vi "AWS Credentials Dialog.vi"(8 "error in (no error)":errorcluster) -> (0 "error out":errorcluster, 2 "Secret Access Key":string="fpHFy/9MTHgVK4Kfo+TPLrNeMAvaW8SEbrhzqAeY", 3 "Access Key ID":string="AKIAZ3CRVRJNHJHHHPO3")   [LabVIEW 2019, in "LV-Data.S3.lvclass"]
uses:
  LV-Data.S3.lvclass
  <vilib>/Platform/browser.llb/Open URL in Default Browser (string).vi
panel:
  in  "Message":string="Please enter your AWS credentials below:"
  in  "OK":bool caption="OK1"
  in  "HELP":bool caption="OK1"
  in  "Secret Access Key":string
  in  "Access Key ID":string
  out "String":string="Please enter your AWS credentials below:"
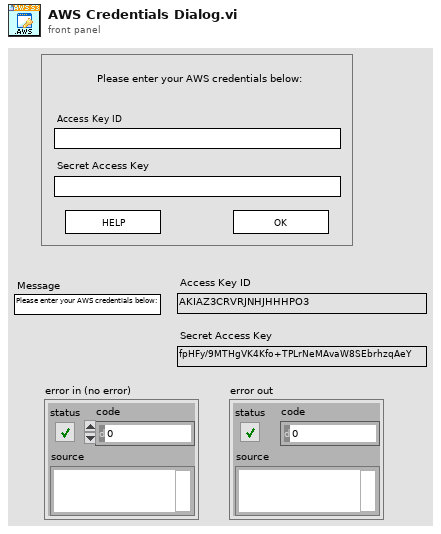
[diagram p1: front panel]
types:
  T1 = enum32{"Invalid", "Standard", "Closed", "Hidden", "Minimized", "Maximized"}
  T2 = enum32{"invalid app kind", "Development System", "Run Time System", "Student Edition", "Embedded LabVIEW", "Evaluation", "Custom"}
  T3 = cluster{"Core":cluster{"Current VI Reference":refnum<vi>, "Close Panel on Exit?":bool}, "Access Key ID":string, "Secret Access Key":string}
  T4 = cluster{"Current VI Reference":refnum<vi>, "Close Panel on Exit?":bool}
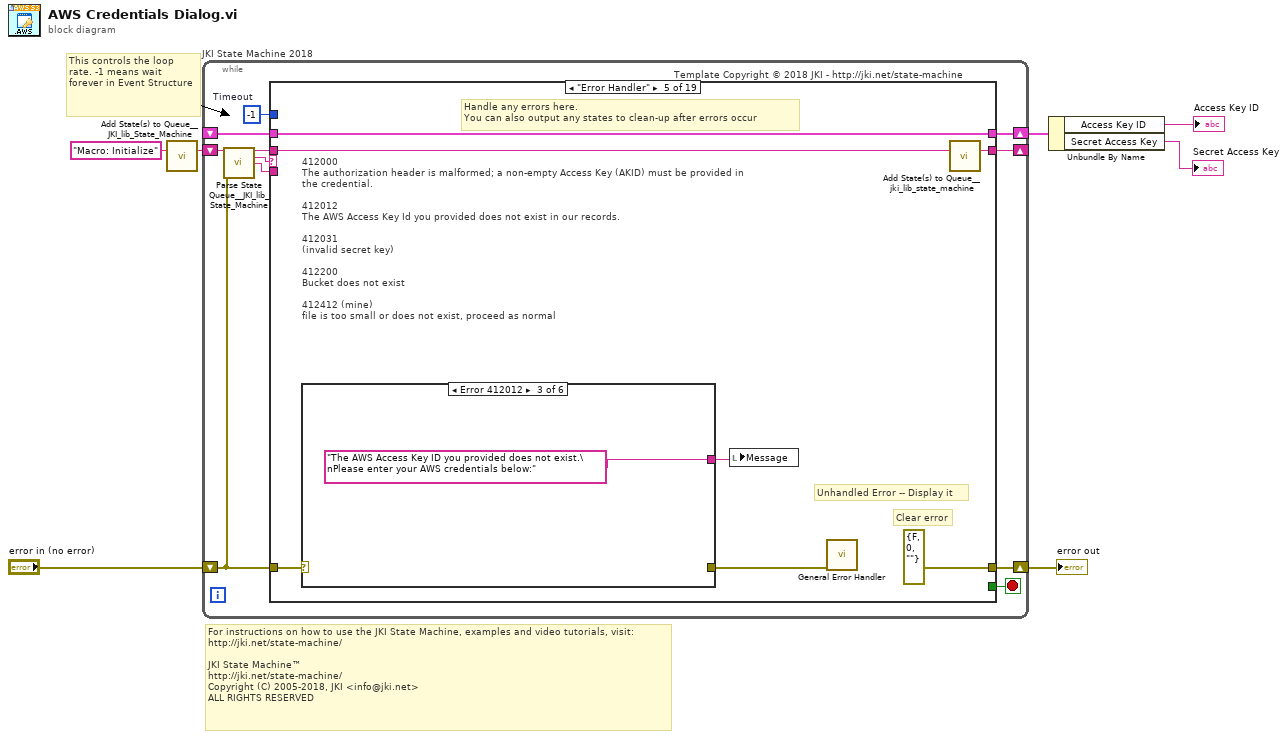
[diagram p0: block diagram]
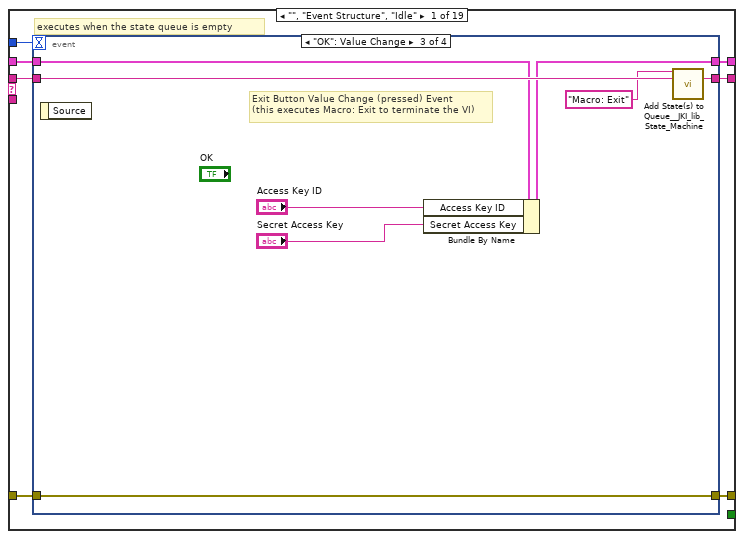
[diagram p2: hidden frame]
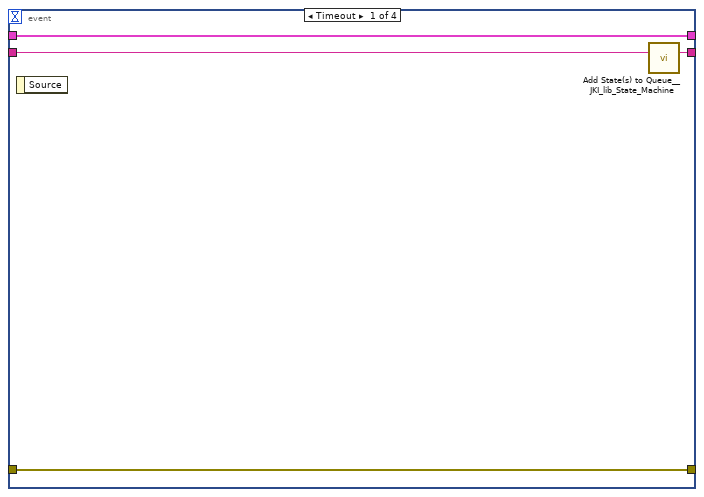
[diagram p3: hidden frame]
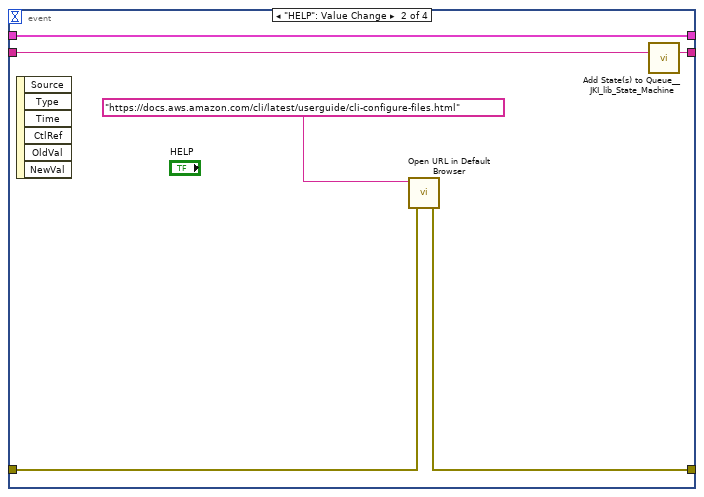
[diagram p4: hidden frame]
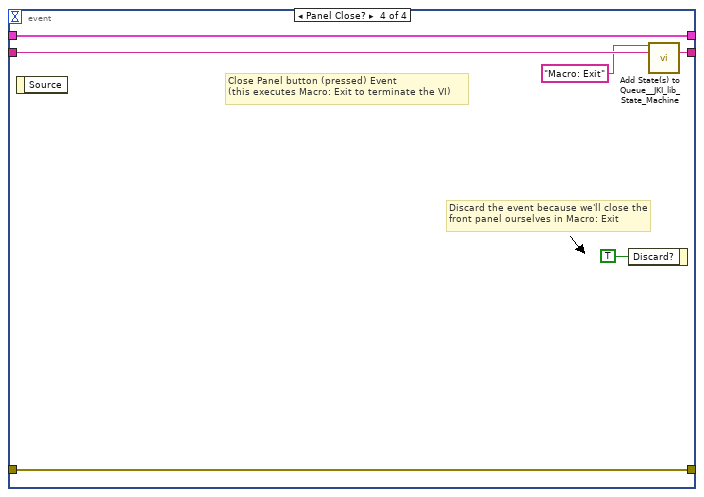
[diagram p5: hidden frame]
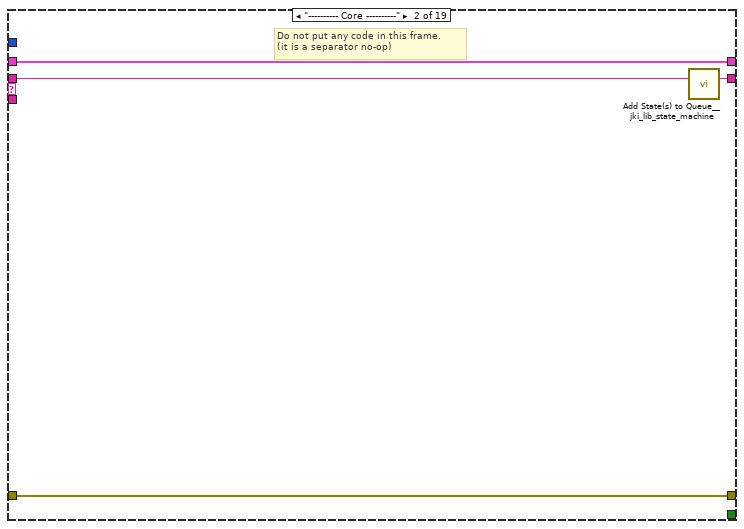
[diagram p6: hidden frame]
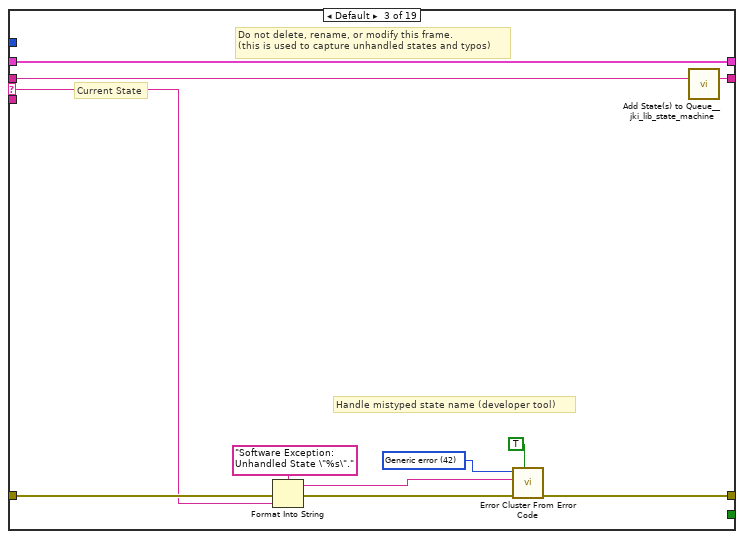
[diagram p7: hidden frame]
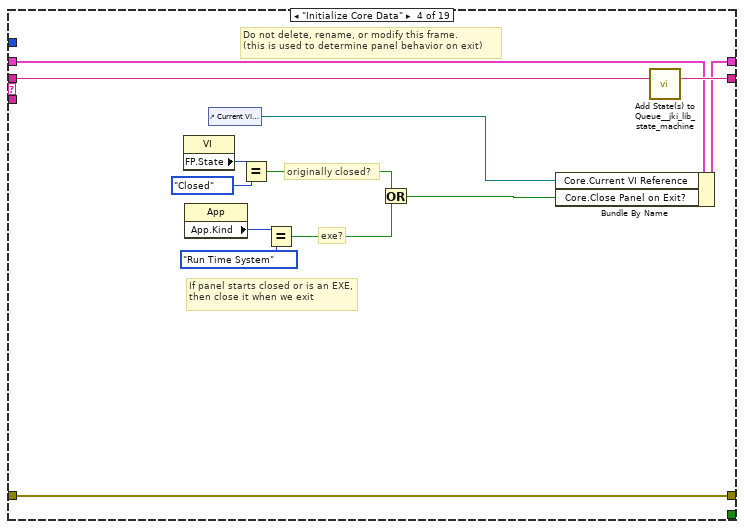
[diagram p8: hidden frame]
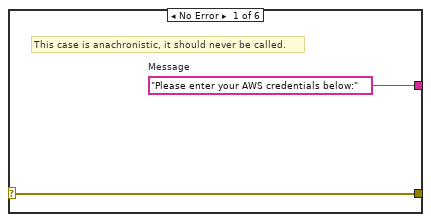
[diagram p9: hidden frame]
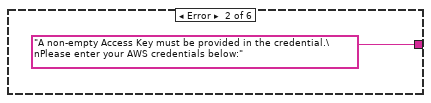
[diagram p10: hidden frame]
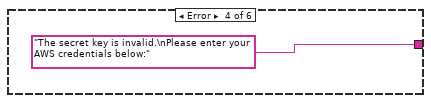
[diagram p11: hidden frame]
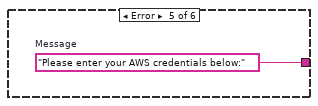
[diagram p12: hidden frame]
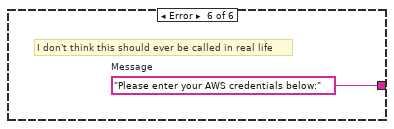
[diagram p13: hidden frame]
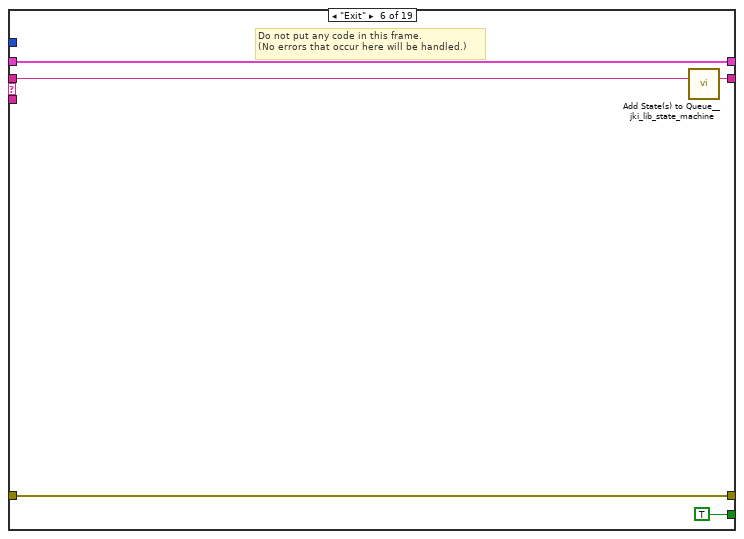
[diagram p14: hidden frame]
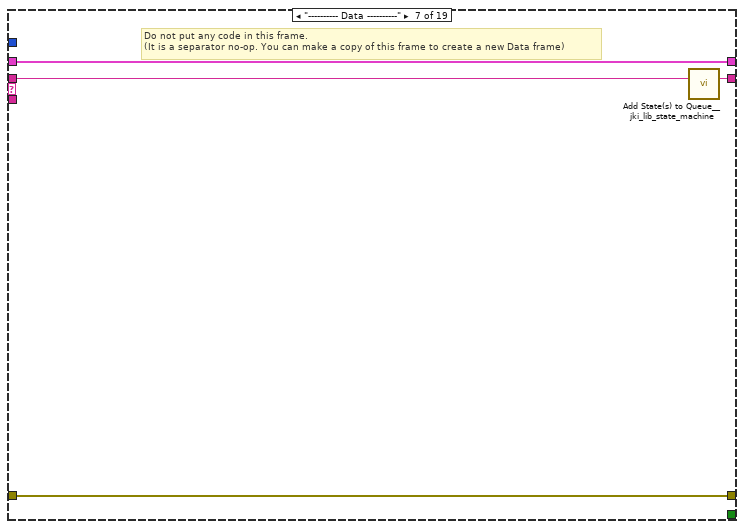
[diagram p15: hidden frame]
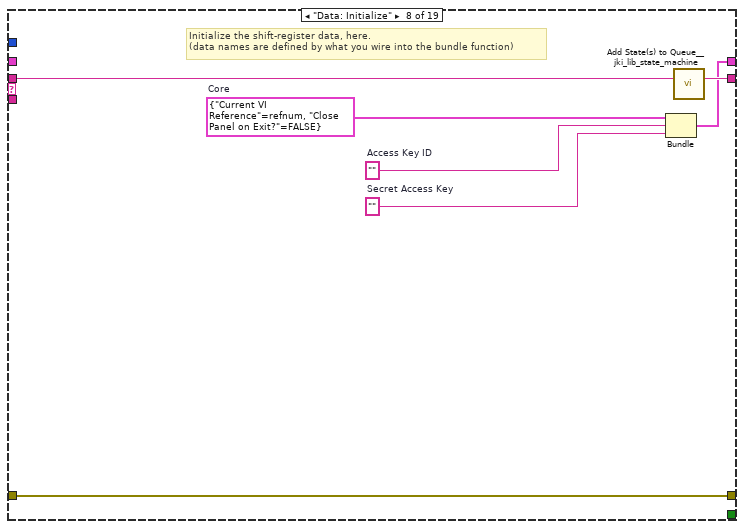
[diagram p16: hidden frame]
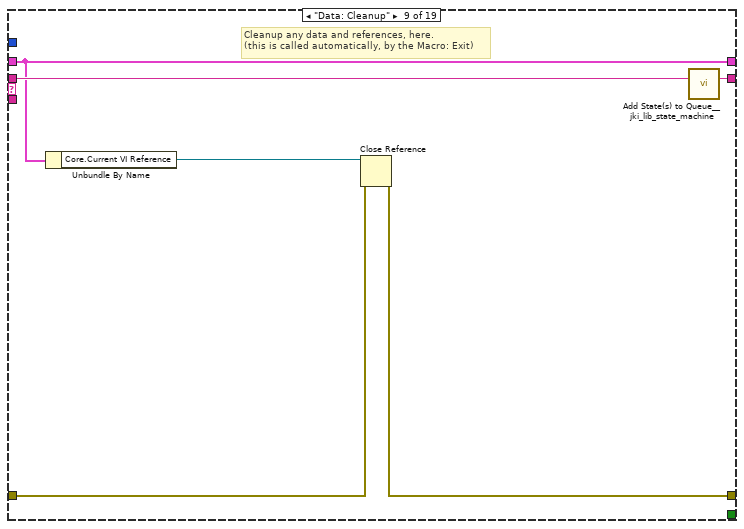
[diagram p17: hidden frame]
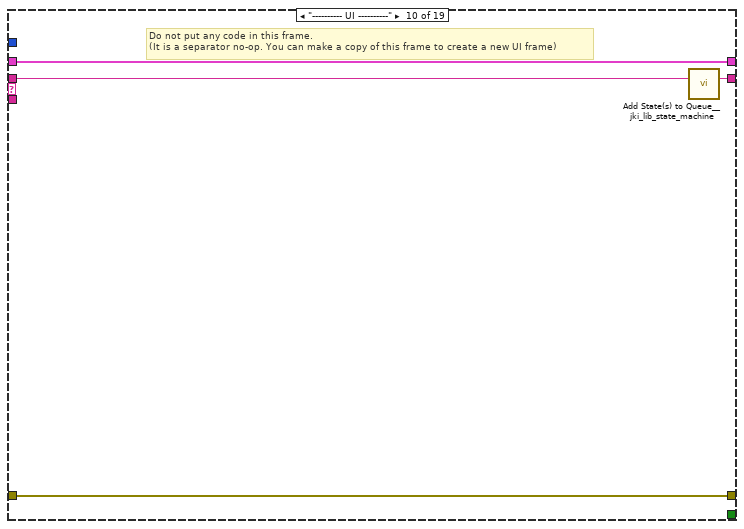
[diagram p18: hidden frame]
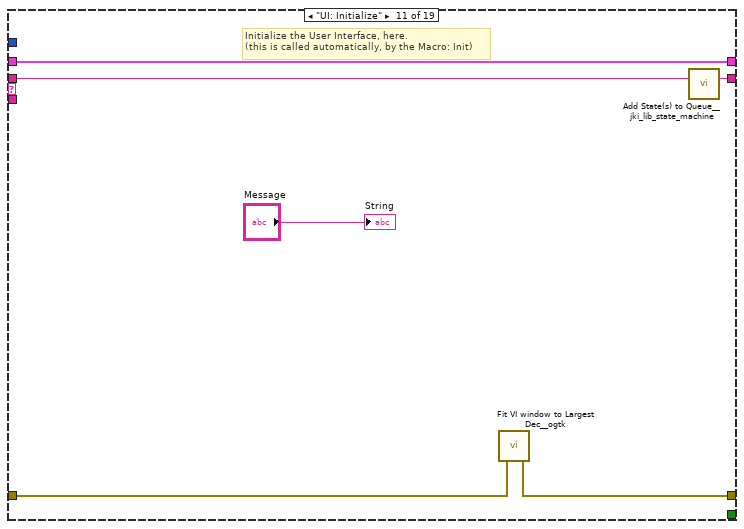
[diagram p19: hidden frame]
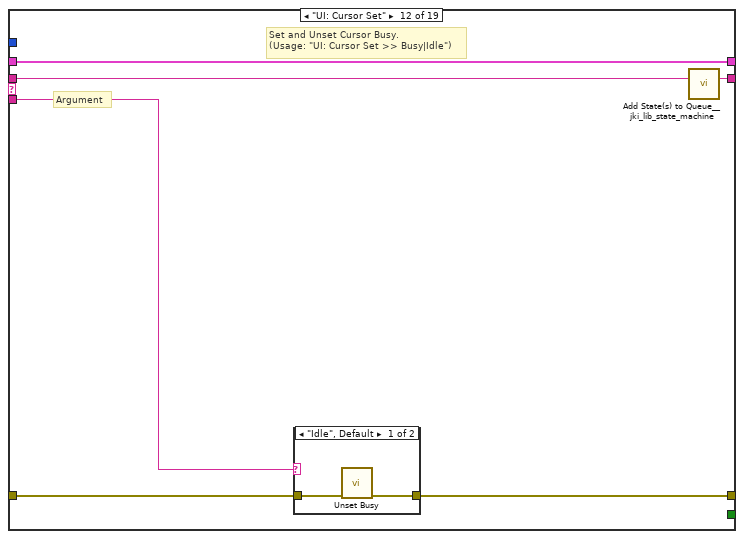
[diagram p20: hidden frame]
diagram:
  # "For instructions on how to use the JKI State Machine, examples and video tutorials, visit:\nhttp://jki.net/state-machine/\n\nJKI State Machine™\nhttp://jki.net/state-machine/\nCopyright (C) 2005-2018, JKI <info@jki.net>\nALL RIGHTS RESERVED"
  # "This controls the loop rate. -1 means wait forever in Event Structure"
  n1 = call <vilib>:"Add State(s) to Queue__JKI_lib_State_Machine.vi"("State(s) in (\"\")"="Macro: Initialize") -> ("States Out"=w7:string)  [unwired: 14 in]
  n2 = while "JKI State Machine 2018" {
    shift-right: [w11] -> w3
    shift-left: _ -> [w10]
    shift-right: [w14] -> w5
    shift-left: "error in (no error)" -> [w8]
    shift-right: [w13] -> _
    shift-left: w7 -> [w15]
    stop <- w12 stop-if-true
    w9 = -1  # Timeout
    # "Template Copyright © 2018 JKI - http://jki.net/state-machine"
    n3 = call <vilib>:"Parse State Queue__JKI_lib_State_Machine.vi"("State Queue"=w15, "Error In (no error)"=w8) -> ("Remaining States"=w17:string, "Current State"=w18:string, "Arguments"=w16:string)  [unwired: 11 in]
    n4 = case shown="\"Error Handler\"" w18 {
      selector: w18 -> [_ _ w54 _ _ _ _ _ _ _ _ _ _ _ _ _ _ _ _]
      tunnel: w17 -> [w25 w53 w58 w77 w84 w96 w100 w107 w113 w117 w123 w129 w140 w209 w214 w224 w228 w232 w236]
      tunnel: w16 -> [_ _ _ _ _ _ _ _ _ _ _ w124 w134 _ _ _ _ _ _]
      tunnel: w10 -> [w23 w50 w56 w70 w78 w94 w97 _ w108 w114 w121 w127 w136 w206 w211 w221 w225 w229 w233]
      tunnel: [w22 w51 w60 w74 errorcluster {"status"=FALSE, "code"=0, "source"=""} ("error out") w93 w98 w104 w109 w115 w119 w125 w137 w207 w212 w222 w226 w230 w234] -> w14
      tunnel: w8 -> [w21 w51 w59 w74 w81 w93 w98 w104 w110 w115 w120 w126 w138 w207 w212 w222 w226 w230 w234]
      tunnel: [w24 w52 w57 w76 w83 w95 w99 w106 w112 w116 w122 w128 w139 w208 w213 w223 w227 w231 w235] -> w13
      tunnel: [_ _ _ _ _ TRUE _ _ _ _ _ _ _ _ _ _ _ _ _] -> w12
      tunnel: [w20 w50 w56 w75 w78 w94 w97 w105 w108 w114 w121 w127 w136 w206 w211 w221 w225 w229 w233] -> w11
      tunnel: w9 -> [w19 _ _ _ _ _ _ _ _ _ _ _ _ _ _ _ _ _ _]
      frame "", "Event Structure", "Idle" {
        # "executes when the state queue is empty"
        n5 = event shown="[2] \"OK\": Value Change" {
          selector: _ -> [_ _ _ _]
          dyn-events: _ -> [_ _ _ _]
          timeout: w19 -> [_ _ _ _]
          tunnel: w25 -> [w29 w35 w43 w49]
          tunnel: [w28 w34 w42 w48] -> w24
          tunnel: w23 -> [w26 w33 w39 w46]
          tunnel: [w27 w31 w41 w47] -> w22
          tunnel: w21 -> [w27 w32 w41 w47]
          tunnel: [w26 w33 w38 w46] -> w20
          event Timeout {
            n6 = event-data() -> ()  [unwired: 1 in, 1 out]
            n7 = call <vilib>:"Add State(s) to Queue__JKI_lib_State_Machine.vi"("State(s) in (\"\")"=w29) -> ("States Out"=w28:string)  [unwired: 14 in]
          }
          event "HELP": Value Change {
            n8 = event-data() -> ()  [unwired: 1 in, 6 out]
            n9 = call-poly <vilib>:"Open URL in Default Browser.vi"("error in (no error)"=w32, "URL"="https://docs.aws.amazon.com/cli/latest/userguide/cli-configure-files.html") -> ("error out"=w31:errorcluster)  [unwired: 4 in, 1 out]
            n10 = call <vilib>:"Add State(s) to Queue__JKI_lib_State_Machine.vi"("State(s) in (\"\")"=w35) -> ("States Out"=w34:string)  [unwired: 14 in]
          }
          event "OK": Value Change {
            # "Exit Button Value Change (pressed) Event\n(this executes Macro: Exit to terminate the VI)"
            n11 = event-data() -> ()  [unwired: 1 in, 1 out]
            n12 = Bundle By Name(cluster=w39, "Access Key ID"="Access Key ID", "Secret Access Key"="Secret Access Key") -> (w38:T3)
            n13 = call <vilib>:"Add State(s) to Queue__JKI_lib_State_Machine.vi"("State(s) in Front (\"\")"="Macro: Exit", "State(s) in (\"\")"=w43) -> ("States Out"=w42:string)  [unwired: 13 in]
          }
          event Panel Close? {
            # "Discard the event because we'll close the front panel ourselves in Macro: Exit"
            # "Close Panel button (pressed) Event\n(this executes Macro: Exit to terminate the VI)"
            n14 = event-data() -> ()  [unwired: 1 in, 1 out]
            n15 = event-data("Discard?"=TRUE) -> ()  [unwired: 1 in, 1 out]
            n16 = call <vilib>:"Add State(s) to Queue__JKI_lib_State_Machine.vi"("State(s) in Front (\"\")"="Macro: Exit", "State(s) in (\"\")"=w49) -> ("States Out"=w48:string)  [unwired: 13 in]
          }
        }
      }
      frame "---------- Core ----------" {
        # "Do not put any code in this frame.\n(it is a separator no-op)"
        n17 = call <vilib>:"Add State(s) to Queue__jki_lib_state_machine.vi"("State(s) in (\"\")"=w53) -> ("States Out"=w52:string)  [unwired: 14 in]
      }
      frame Default {
        w63 = 42 items=["No error", "Argument error", "Memory is full", "Out of zone", "End of file", "File already open", "Generic file I/O error", "File not found", "File permission error", "Disk is full", "Duplicate path", "Too many files open", "System feature not enabled", "Resource file not found", "Cannot add resource", "Resource not found", "Image not found", "Image memory error", "Pen does not exist", "Config type invalid", "Config token not found", "Config parse error", "Config memory error", "Bad external code format", "Bad external code offset", "External code not present", "Null window", "Destroy window error", "Null menu", "Print aborted", "Bad print record", "Print driver error", "Windows error during printing", "Memory error during printing", "Print dialog error", "Generic print error", "Invalid device refnum", "Device not found", "Device parameter error", "Device unit error", "Cannot open device", "Device call aborted", "Generic error", "Cancelled by user", "Object ID too low", "Object ID too high", "Object not in heap", "Unknown heap", "Unknown object (invalid DefProc)", "Unknown object (DefProc not in table)", "Message out of range", "Invalid (null) method", "Unknown message", "Manager call not supported", "Bad address", "Network operation in progress", "Network operation timed out", "Connection is busy", "Network attribute not supported", "Network error", "Address in use", "System out of memory", "Connection aborted", "Connection refused", "Not connected", "Already connected", "Connection closed", "Initialization error (interapplication manager)", "Bad occurrence", "Wait on unbound occurrence handler", "Occurrence queue overflow", "Datalog type conflict", "Unused", "Unrecognized type (interapplication manager)", "Memory corrupt", "Failed to make temporary DLL", "Old CIN version", "Drag socket not found", "Failed to load drop-object", "Failed to register OLE object", "Failed to release OLE object", "Format specifier type mismatch", "Unknown format specifier", "Too few format specifiers", "Too many format specifiers", "Scan failed", "Newer CIN version", "Error converting to variant", "Runtime menu error", "Password tampered", "Variant attribute not found", "Incompatible variant data type", "Event data is not available", "Event Store is not present", "Occurrence is not found", "Event Queue is not created", "Event info is not available", "Refnum passed is NULL", "Error retrieving Class GUID", "Error retrieving CoClass GUID", "Error retrieving TypeLib GUID.", "Bad built application magic bytes.", "Specific driver is different from the specific driver associated with the Logical Name.", "There is no session opened to the class driver.", "Max Error", "MAX - Error with config objects", "MAX - Error loading configuration", "MAX - Group not supported"]
        # "Current State"
        # "Do not delete, rename, or modify this frame.\n(this is used to capture unhandled states and typos)"
        # "Handle mistyped state name (developer tool)"
        n18 = Format Into String(format string="Software Exception: Unhandled State \"%s\"." ("message"), error in=w59, w54) -> (resulting string=w62:string, error out=w61:errorcluster)  [unwired: 1 in]
        n19 = call <vilib>:"Error Cluster From Error Code.vi"("show call chain? (False)"=TRUE, "error in (no error)"=w61, "error message (\"\")"=w62, "error code (0)"=w63) -> ("error out"=w60:errorcluster)  [unwired: 5 in]
        n20 = call <vilib>:"Add State(s) to Queue__jki_lib_state_machine.vi"("State(s) in (\"\")"=w58) -> ("States Out"=w57:string)  [unwired: 14 in]
      }
      frame "Initialize Core Data" {
        # "Do not delete, rename, or modify this frame.\n(this is used to determine panel behavior on exit)"
        # "originally closed?"
        # "exe?"
        # "If panel starts closed or is an EXE, then close it when we exit"
        n21 = property class="VI"() -> ("FP.State"=w67:T1)  [unwired: 2 in, 2 out]
        n22 = property class="App"() -> ("App.Kind"=w73:T2)  [unwired: 2 in, 2 out]
        n23 = control-ref of="Current VI Reference"() -> (w68:refnum<vi>)
        n24 = Equal?(x=w67, y=T1."Closed" ("Front Panel Window:State")) -> (x = y?=w65:bool)
        n25 = Equal?(x=w73, y=T2."Run Time System" ("Application:Kind")) -> (x = y?=w71:bool)
        n26 = Or(x=w65, y=w71) -> (x .or. y?=w69:bool)
        n27 = Bundle By Name(cluster=w70, "Core.Current VI Reference"=w68, "Core.Close Panel on Exit?"=w69) -> (w75:T3)
        n28 = call <vilib>:"Add State(s) to Queue__jki_lib_state_machine.vi"("State(s) in (\"\")"=w77) -> ("States Out"=w76:string)  [unwired: 14 in]
      }
      frame "Error Handler" {
        # "412000\nThe authorization header is malformed; a non-empty Access Key (AKID) must be provided in the credential.\n\n412012\nThe AWS Access Key Id you provided does not exist in our records.\n\n412031\n(invalid secret key)\n\n412200\nBucket does not exist\n\n412412 (mine)\nfile is too small or does not exist, proceed as normal"
        # "Unhandled Error -- Display it"
        # "Handle any errors here.\nYou can also output any states to clean-up after errors occur"
        # "Clear error"
        n29 = case shown="Error 412012" w81 {
          selector: w81 -> [w86 _ _ _ _ _]
          tunnel: [w86 _ _ _ _ _] -> w80
          tunnel: [w85 "A non-empty Access Key must be provided in the credential.\nPlease enter your AWS credentials below:" "The AWS Access Key ID you provided does not exist.\nPlease enter your AWS credentials below:" "The secret key is invalid.\nPlease enter your AWS credentials below:" w90 w91] -> w79
          frame No Error {
            w85 = "Please enter your AWS credentials below:"  # Message
            # "This case is anachronistic, it should never be called."
          }
          frame Error {
          }
          frame Error {
          }
          frame Error {
          }
          frame Error {
            w90 = "Please enter your AWS credentials below:"  # Message
          }
          frame Error {
            w91 = "Please enter your AWS credentials below:"  # Message
            # "I don't think this should ever be called in real life"
          }
        }
        n30 = local write "Message"(w79) -> ()
        n31 = call <vilib>:"General Error Handler.vi"("error in (no error)"=w80) -> ()  [unwired: 10 in, 5 out]
        n32 = call <vilib>:"Add State(s) to Queue__jki_lib_state_machine.vi"("State(s) in (\"\")"=w84) -> ("States Out"=w83:string)  [unwired: 14 in]
      }
      frame "Exit" {
        # "Do not put any code in this frame.\n(No errors that occur here will be handled.)"
        n33 = call <vilib>:"Add State(s) to Queue__jki_lib_state_machine.vi"("State(s) in (\"\")"=w96) -> ("States Out"=w95:string)  [unwired: 14 in]
      }
      frame "---------- Data ----------" {
        # "Do not put any code in this frame.\n(It is a separator no-op. You can make a copy of this frame to create a new Data frame)"
        n34 = call <vilib>:"Add State(s) to Queue__jki_lib_state_machine.vi"("State(s) in (\"\")"=w100) -> ("States Out"=w99:string)  [unwired: 14 in]
      }
      frame "Data: Initialize" {
        w101 = ""  # Access Key ID
        w102 = T4 {"Current VI Reference"=refnum, "Close Panel on Exit?"=FALSE}  # Core
        w103 = ""  # Secret Access Key
        # "Initialize the shift-register data, here.\n(data names are defined by what you wire into the bundle function)"
        n35 = Bundle("Core"=w102, "Access Key ID"=w101, "Secret Access Key"=w103) -> (w105:T3)  [unwired: 1 in]
        n36 = call <vilib>:"Add State(s) to Queue__jki_lib_state_machine.vi"("State(s) in (\"\")"=w107) -> ("States Out"=w106:string)  [unwired: 14 in]
      }
      frame "Data: Cleanup" {
        # "Cleanup any data and references, here.\n(this is called automatically, by the Macro: Exit)"
        n37 = Unbundle By Name(w108) -> ("Core.Current VI Reference"=w111:refnum<vi>)
        n38 = Close Reference(reference=w111, error in (no error)=w110) -> (error out=w109:errorcluster)
        n39 = call <vilib>:"Add State(s) to Queue__jki_lib_state_machine.vi"("State(s) in (\"\")"=w113) -> ("States Out"=w112:string)  [unwired: 14 in]
      }
      frame "---------- UI ----------" {
        # "Do not put any code in this frame.\n(It is a separator no-op. You can make a copy of this frame to create a new UI frame)"
        n40 = call <vilib>:"Add State(s) to Queue__jki_lib_state_machine.vi"("State(s) in (\"\")"=w117) -> ("States Out"=w116:string)  [unwired: 14 in]
      }
      frame "UI: Initialize" {
        # "Initialize the User Interface, here.\n(this is called automatically, by the Macro: Init)"
        n41 = call <userlib>:"Fit VI window to Largest Dec__ogtk.vi"("error in (no error)"=w120) -> ("error out"=w119:errorcluster)  [unwired: 5 in, 1 out]
        n42 = call <vilib>:"Add State(s) to Queue__jki_lib_state_machine.vi"("State(s) in (\"\")"=w123) -> ("States Out"=w122:string)  [unwired: 14 in]
        "String" <- "Message"
      }
      frame "UI: Cursor Set" {
        # "Argument"
        # "Set and Unset Cursor Busy.\n(Usage: \"UI: Cursor Set >> Busy|Idle\")"
        n43 = case shown="\"Idle\", Default" w124 {
          tunnel: w126 -> [w131 w133]
          tunnel: [w130 w132] -> w125
          frame "Idle", Default {
            n44 = call <vilib>:"Unset Busy.vi"("error in (no error)"=w131) -> ("error out"=w130:errorcluster)  [unwired: 10 in]
          }
          frame "Busy" {
            n45 = call <vilib>:"Set Busy.vi"("error in (no error)"=w133) -> ("error out"=w132:errorcluster)  [unwired: 9 in, 1 out]
          }
        }
        n46 = call <vilib>:"Add State(s) to Queue__jki_lib_state_machine.vi"("State(s) in (\"\")"=w129) -> ("States Out"=w128:string)  [unwired: 14 in]
      }
      frame "UI: Front Panel State" {
        # "Argument"
        # "Set Front Panel Open or Closed\n(Usage: \"UI: Front Panel State >> Open|Close\")"
        n47 = Unbundle By Name(w136) -> ("Core.Current VI Reference"=w135:refnum<vi>)
        n48 = case shown="\"Open\", \"Standard\", Default" w134 {
          tunnel: w138 -> [w146 w161 w172 w185 w198]
          tunnel: [w148 w162 w174 w187 w200] -> w137
          tunnel: w135 -> [w147 w159 w173 w186 w199]
          frame "Open", "Standard", Default {
            w141 = T1."Standard" ("State")
            n49 = property class="VI"(reference=w147, error in=w146) -> (reference out=w144:refnum<vi>, error out=w145:errorcluster, "FP.State"=w143:T1)
            n50 = Not Equal?(x=w143, y=w141) -> (x != y?=w142:bool)
            n51 = case shown="False" w142 {
              tunnel: [w152 w154] -> w148
              tunnel: w145 -> [w151 w154]
              tunnel: w144 -> [w150 _]
              tunnel: w141 -> [w149 _]
              frame True {
                n52 = invoke class="VI" method="FP.Open"(reference=w150, error in=w151, "Activate"=TRUE, "State"=w149) -> (error out=w152:errorcluster)  [unwired: 1 in, 4 out]
              }
              frame False {
              }
            }
          }
          frame "Close", "Closed" {
            n53 = property class="VI"(reference=w159, error in=w161) -> (reference out=w158:refnum<vi>, error out=w160:errorcluster, "FP.State"=w156:T1)
            n54 = Not Equal?(x=w156, y=T1."Closed" ("Front Panel Window:State")) -> (x != y?=w155:bool)
            n55 = case shown="True" w155 {
              tunnel: [w163 w166] -> w162
              tunnel: w160 -> [w163 w165]
              tunnel: w158 -> [_ w164]
              frame False {
              }
              frame True {
                n56 = invoke class="VI" method="FP.Close"(reference=w164, error in=w165) -> (error out=w166:errorcluster)  [unwired: 1 in, 2 out]
              }
            }
          }
          frame "Hidden", "Hide" {
            w167 = T1."Hidden" ("State")
            n57 = property class="VI"(reference=w173, error in=w172) -> (reference out=w170:refnum<vi>, error out=w171:errorcluster, "FP.State"=w169:T1)
            n58 = Not Equal?(x=w169, y=w167) -> (x != y?=w168:bool)
            n59 = case shown="True" w168 {
              tunnel: [w178 w179] -> w174
              tunnel: w171 -> [w177 w179]
              tunnel: w170 -> [w176 _]
              tunnel: w167 -> [w175 _]
              frame True {
                n60 = invoke class="VI" method="FP.Open"(reference=w176, error in=w177, "State"=w175) -> (error out=w178:errorcluster)  [unwired: 2 in, 4 out]
              }
              frame False {
              }
            }
          }
          frame "Minimize", "Minimized" {
            w180 = T1."Minimized" ("State")
            n61 = property class="VI"(reference=w186, error in=w185) -> (reference out=w183:refnum<vi>, error out=w184:errorcluster, "FP.State"=w182:T1)
            n62 = Not Equal?(x=w182, y=w180) -> (x != y?=w181:bool)
            n63 = case shown="True" w181 {
              tunnel: [w191 w192] -> w187
              tunnel: w184 -> [w190 w192]
              tunnel: w183 -> [w189 _]
              tunnel: w180 -> [w188 _]
              frame True {
                n64 = invoke class="VI" method="FP.Open"(reference=w189, error in=w190, "State"=w188) -> (error out=w191:errorcluster)  [unwired: 2 in, 4 out]
              }
              frame False {
              }
            }
          }
          frame "Maximize", "Maximized" {
            w193 = T1."Maximized" ("State")
            n65 = property class="VI"(reference=w199, error in=w198) -> (reference out=w196:refnum<vi>, error out=w197:errorcluster, "FP.State"=w195:T1)
            n66 = Not Equal?(x=w195, y=w193) -> (x != y?=w194:bool)
            n67 = case shown="True" w194 {
              tunnel: [w204 w205] -> w200
              tunnel: w197 -> [w203 w205]
              tunnel: w196 -> [w202 _]
              tunnel: w193 -> [w201 _]
              frame True {
                n68 = invoke class="VI" method="FP.Open"(reference=w202, error in=w203, "State"=w201) -> (error out=w204:errorcluster)  [unwired: 2 in, 4 out]
              }
              frame False {
              }
            }
          }
        }
        n69 = call <vilib>:"Add State(s) to Queue__jki_lib_state_machine.vi"("State(s) in (\"\")"=w140) -> ("States Out"=w139:string)  [unwired: 14 in]
      }
      frame "---------- Macro ----------" {
        # "Do not put any code in this frame.\n(It is a separator no-op. You can make a copy of this frame to create a new Macro frame)"
        n70 = call <vilib>:"Add State(s) to Queue__jki_lib_state_machine.vi"("State(s) in (\"\")"=w209) -> ("States Out"=w208:string)  [unwired: 14 in]
      }
      frame "Macro: Initialize" {
        w210 = "Data: Initialize\nInitialize Core Data\nUI: Initialize\nUI: Front Panel State >> Open"  # Data: Initialize Initialize Core Data UI: Initialize UI: Front Panel State >> Open
        # "Initialization Macro\n(This is called once, when the VI starts)"
        n71 = call <vilib>:"Add State(s) to Queue__jki_lib_state_machine.vi"("State(s) in Front (\"\")"=w210, "State(s) in (\"\")"=w214) -> ("States Out"=w213:string)  [unwired: 13 in]
      }
      frame "Macro: Exit" {
        # "Exit Macro\n(This is called once, when the VI exits)"
        n72 = Unbundle By Name(w221) -> ("Core.Close Panel on Exit?"=w220:bool)
        n73 = Select(t="UI: Front Panel State >> Close", s=w220, f="") -> (s? t:f=w217:string)
        n74 = call <vilib>:"Add State(s) to Queue__jki_lib_state_machine.vi"("State(s) in (\"\")"=w217, "State(s) at Back (\"\")"="Data: Cleanup\nExit") -> ("States Out"=w215:string)  [unwired: 13 in]
        n75 = call <vilib>:"Add State(s) to Queue__jki_lib_state_machine.vi"("State(s) in Front (\"\")"=w215, "State(s) in (\"\")"=w224) -> ("States Out"=w223:string)  [unwired: 13 in]
      }
      frame "---------- New Category ----------" {
        # "Template Separator\n(You can make a copy of, or modify, this frame)"
        n76 = call <vilib>:"Add State(s) to Queue__jki_lib_state_machine.vi"("State(s) in (\"\")"=w228) -> ("States Out"=w227:string)  [unwired: 14 in]
      }
      frame "New Category: 1" {
        # "Your code here.\n(You can make a copy of, or modify, this frame)"
        n77 = call <vilib>:"Add State(s) to Queue__jki_lib_state_machine.vi"("State(s) in (\"\")"=w232) -> ("States Out"=w231:string)  [unwired: 14 in]
      }
      frame "New Category: 2" {
        # "Your code here.\n(You can make a copy of, or modify, this frame)"
        n78 = call <vilib>:"Add State(s) to Queue__jki_lib_state_machine.vi"("State(s) in (\"\")"=w236) -> ("States Out"=w235:string)  [unwired: 14 in]
      }
    }
  }
  "error out" <- w5
  n79 = Unbundle By Name(w3) -> ("Access Key ID"=→"Access Key ID":string, "Secret Access Key"=→"Secret Access Key":string)
